vi "Set Drive Motors.vi"(5 "Disable":bool, 6 "Drive PID Slot":i32, 7 "Max Velocity(RPM)":dbl=200.0, 8 "Drive Control Mode":T11, 9 "Motor List":T1[](array[typedef])=[enum."Right-Front", enum."Left-Front", enum."Left-Back", enum."Right-Back"], 10 "Swerve Data":T2 {"Back Right"."Angle" scale format="%.3f"; "Back Right"."Velocity" scale=-1.0..1.0 scale format="%.1f"; "Back Left"."Angle" scale format="%.3f"; "Back Left"."Velocity" scale=-1.0..1.0 scale format="%.1f"; "Front Left"."Angle" scale format="%.3f"; "Front Left"."Velocity" scale=-1.0..1.0 scale format="%.1f"; "Front Right"."Angle" scale format="%.3f"; "Front Right"."Velocity" scale=-1.0..1.0 scale format="%.1f"}, 11 "Drive Refs":T6[](array[typedef])) -> (1 "Speeds":dbl[](array[numeric]), 3 "Array Out":T6[](array[typedef]))   [LabVIEW 2023, in "TShirtWork-SwerveDrive_ACT_ts.lvlib"]
uses:
  TShirtWork-SwerveDrive_ACT_ts.lvlib
  <vilib>/Rock Robotics/SystemInterfaces/DIO/FPGA_DIOPWMChannel.ctl
  <vilib>/Rock Robotics/WPI/PWM/WPI_PWMDeadband.ctl
  <vilib>/Rock Robotics/WPI/MotorControl/WPI_MotorControlType.ctl
  <vilib>/Rock Robotics/SystemInterfaces/DIO/FPGA_DIOChannel.ctl
  <vilib>/Rock Robotics/WPI/MotorControl/WPI_MotorControlDeviceRef.ctl
  <vilib>/Rock Robotics/WPI/ThirdParty/REV Robotics/REVLib/Typedef/Spark MAX Control Type.ctl
  Shared Code/TypeDefs/Level_Velocity plus-minus 1.ctl
  Shared Code/TypeDefs/Dial_Compase heading unit circle CCW positive.ctl
  Shared Code/TypeDefs/Cluster_Module Velocity-Direction-Rotations.ctl
  Shared Code/TypeDefs/Cluster_Swerve 4 Steer and Velocity.ctl
  Shared Code/TypeDefs/ENUM_Module Position.ctl
panel:
  # "\"Front\" of Robot"
  # "Right Hand Rule"
  # "X"
  # "+CCW"
  # "Y"
  # "(0,0)"
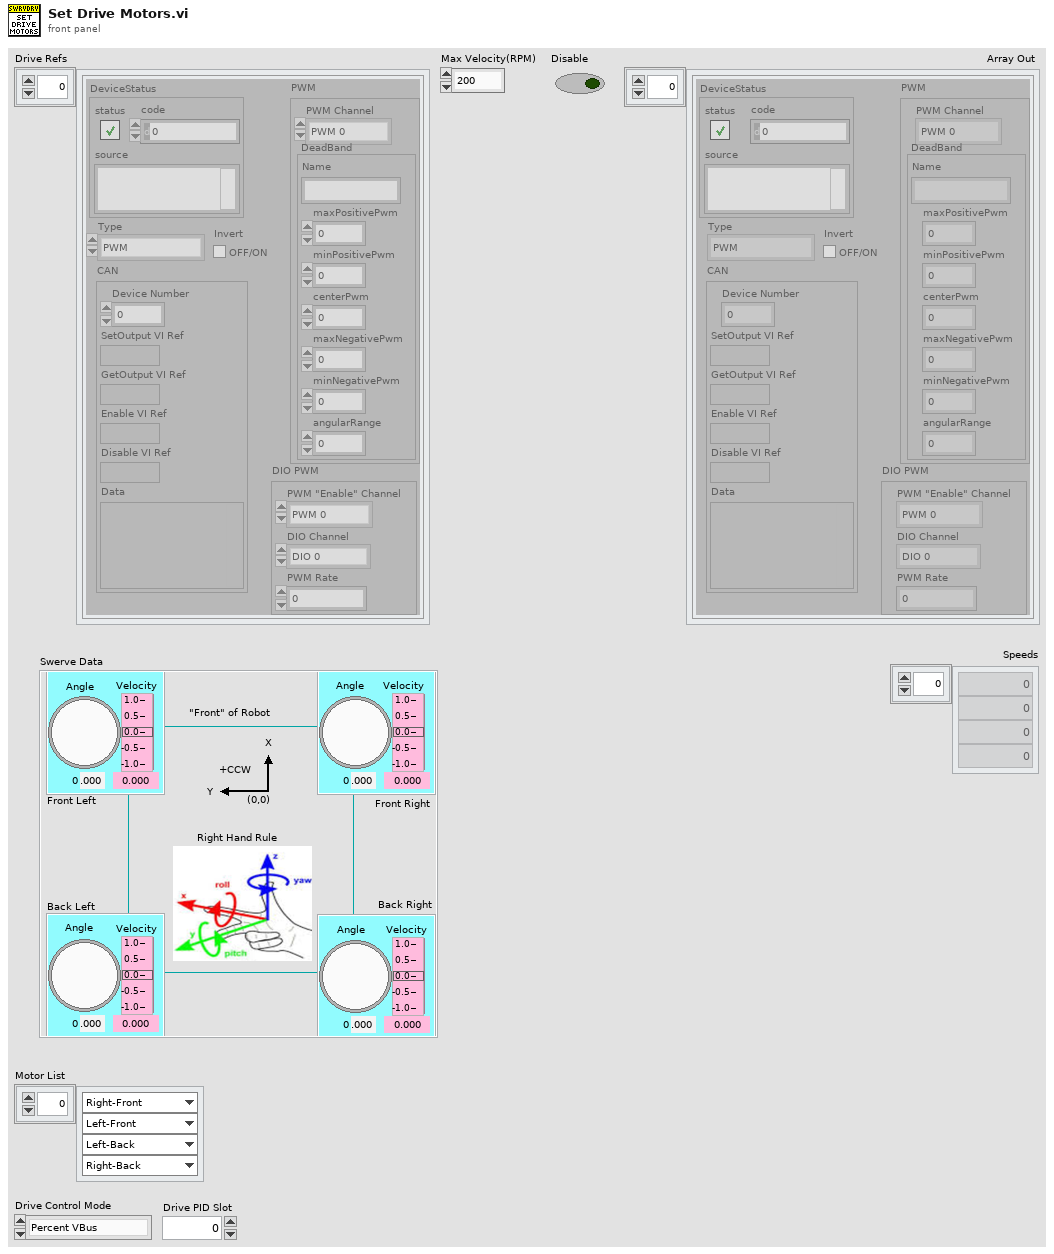
[diagram p1: front panel]
types:
  T1 = typedef "ENUM_Module Position.ctl" = enum16{"Left-Front", "Right-Front", "Left-Back", "Right-Back"}
  T2 = typedef "Cluster_Swerve 4 Steer and Velocity.ctl" = cluster{"Front Right":T3, "Front Left":T3, "Back Left":T3, "Back Right":T3}
  T3 = typedef "Cluster_Module Velocity-Direction-Rotations.ctl" = cluster{"Velocity":T4, "Angle":T5, "Rotations Count":dbl}
  T4 = typedef "Level_Velocity plus-minus 1.ctl" = dbl
  T5 = typedef "Dial_Compase heading unit circle CCW positive.ctl" = dbl
  T6 = typedef "WPI_MotorControlDeviceRef.ctl" = cluster{"DeviceStatus":errorcluster, "Type":T7, "PWM":cluster{"PWM Channel":T8, "DeadBand":T9}, "CAN":cluster{"Device Number":u8, "SetOutput VI Ref":variant, "GetOutput VI Ref":variant, "Enable VI Ref":variant, "Disable VI Ref":variant, "Data":variant}, "Invert":bool, "DIO PWM":cluster{"PWM \"Enable\" Channel":T8, "DIOChannel":T10, "PWM Rate":dbl}}
  T7 = typedef "WPI_MotorControlType.ctl" = enum16{"PWM", "CAN", "DIO PWM"}
  T8 = typedef "FPGA_DIOPWMChannel.ctl" = enum8{"PWM 0", "PWM 1", "PWM 2", "PWM 3", "PWM 4", "PWM 5", "PWM 6", "PWM 7", "PWM 8", "PWM 9", "PWM MXP 0", "PWM MXP 1", "PWM MXP 2", "PWM MXP 3", "PWM MXP 4", "PWM MXP 5", "PWM MXP 6", "PWM MXP 7", "PWM MXP 8", "PWM MXP 9", "Invalid"}
  T9 = typedef "WPI_PWMDeadband.ctl" = cluster{"Name":string, "maxPositivePwm":i32, "minPositivePwm":i32, "centerPwm":i32, "maxNegativePwm":i32, "minNegativePwm":i32, "angularRange":u16}
  T10 = typedef "FPGA_DIOChannel.ctl" = enum8{"DIO 0", "DIO 1", "DIO 2", "DIO 3", "DIO 4", "DIO 5", "DIO 6", "DIO 7", "DIO 8", "DIO 9", "DIO MXP 0", "DIO MXP 1", "DIO MXP 2", "DIO MXP 3", "DIO MXP 4", "DIO MXP 5", "DIO MXP 6", "DIO MXP 7", "DIO MXP 8", "DIO MXP 9", "DIO MXP 10", "DIO MXP 11", "DIO MXP 12", "DIO MXP 13", "DIO MXP 14", "DIO MXP 15", "SPI Port CS1", "SPI Port CS2", "SPI Port CS3", "SPI Port MISO", "SPI Port MOSI", "Invalid"}
  T11 = typedef "Spark MAX Control Type.ctl" = enum16{"Percent VBus", "Voltage", "Velocity", "Position", "Smart Motion", "Current", "Smart Velocity"}
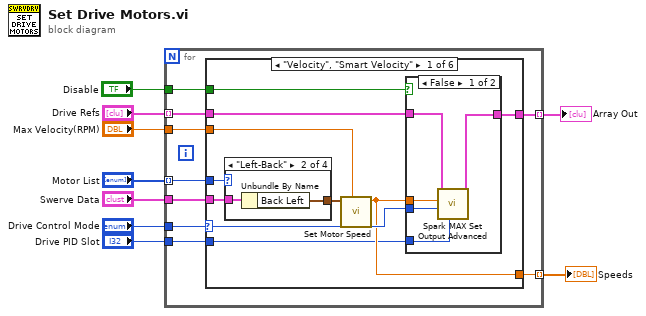
[diagram p0: block diagram]
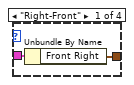
[diagram p3: hidden frame]
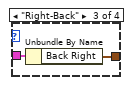
[diagram p4: hidden frame]
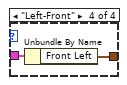
[diagram p5: hidden frame]
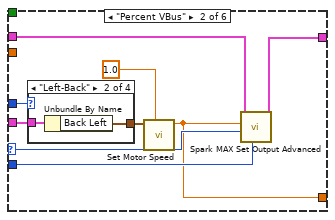
[diagram p6: hidden frame]
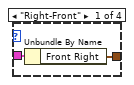
[diagram p7: hidden frame]
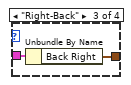
[diagram p8: hidden frame]
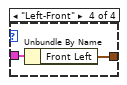
[diagram p9: hidden frame]
diagram:
  n1 = for {
    tunnel: "Drive Refs" -> [w18] mode=indexing
    tunnel: "Drive Control Mode" -> [w17]
    tunnel: "Drive PID Slot" -> [w16]
    tunnel: [w15] -> w9 mode=indexing
    tunnel: "Max Velocity(RPM)" -> [w12]
    tunnel: "Motor List" -> [w14] mode=indexing
    tunnel: "Swerve Data" -> [w13]
    tunnel: [w11] -> w2 mode=indexing
    tunnel: "Disable" -> [w10]
    n2 = case shown="\"Velocity\", \"Smart Velocity\"" w17 {
      selector: w17 -> [w27 w50 _ _ _ _]
      tunnel: w18 -> [w28 w51 w60 w61 w62 w63]
      tunnel: w16 -> [w20 w49 _ _ _ _]
      tunnel: [w26 w48 w60 w61 w62 w63] -> w15
      tunnel: w14 -> [w24 w46 _ _ _ _]
      tunnel: w13 -> [w25 w47 _ _ _ _]
      tunnel: w12 -> [w22 _ _ _ _ _]
      tunnel: [w21 w43 _ _ _ _] -> w11
      tunnel: w10 -> [w19 _ _ _ _ _]
      frame "Velocity", "Smart Velocity" {
        n3 = case shown="\"Left-Back\"" w24 {
          tunnel: w25 -> [w36 w38 w40 w42]
          tunnel: [w35 w37 w39 w41] -> w23
          frame "Right-Front" {
            n4 = Unbundle By Name(w36) -> ("Front Right"=w35:T3)
          }
          frame "Left-Back" {
            n5 = Unbundle By Name(w38) -> ("Back Left"=w37:T3)
          }
          frame "Right-Back" {
            n6 = Unbundle By Name(w40) -> ("Back Right"=w39:T3)
          }
          frame "Left-Front" {
            n7 = Unbundle By Name(w42) -> ("Front Left"=w41:T3)
          }
        }
        n8 = call "Set Motor Speed.vi"("Max Velocity"=w22, "Front Left"=w23) -> ("Velocity Value Set Out"=w21:dbl)  [unwired: 9 in]
        n9 = case shown="False" w19 {
          tunnel: w28 -> [w33 w34]
          tunnel: w27 -> [w32 _]
          tunnel: [w31 w34] -> w26
          tunnel: w21 -> [w30 _]
          tunnel: w20 -> [w29 _]
          frame False {
            n10 = call <vilib>:"Spark MAX Set Output Advanced.vi"("PIDF Slot (0)"=w29, "Control Mode"=w32, "Setpoint"=w30, "MotorControlDevRef"=w33) -> ("MotorControlDevRef"=w31:T6)  [unwired: 6 in, 1 out]
          }
          frame True {
          }
        }
      }
      frame "Percent VBus" {
        n11 = case shown="\"Left-Back\"" w46 {
          tunnel: w47 -> [w53 w55 w57 w59]
          tunnel: [w52 w54 w56 w58] -> w45
          frame "Right-Front" {
            n12 = Unbundle By Name(w53) -> ("Front Right"=w52:T3)
          }
          frame "Left-Back" {
            n13 = Unbundle By Name(w55) -> ("Back Left"=w54:T3)
          }
          frame "Right-Back" {
            n14 = Unbundle By Name(w57) -> ("Back Right"=w56:T3)
          }
          frame "Left-Front" {
            n15 = Unbundle By Name(w59) -> ("Front Left"=w58:T3)
          }
        }
        n16 = call "Set Motor Speed.vi"("Max Velocity"=1.0, "Front Left"=w45) -> ("Velocity Value Set Out"=w43:dbl)  [unwired: 9 in]
        n17 = call <vilib>:"Spark MAX Set Output Advanced.vi"("PIDF Slot (0)"=w49, "Control Mode"=w50, "Setpoint"=w43, "MotorControlDevRef"=w51) -> ("MotorControlDevRef"=w48:T6)  [unwired: 6 in, 1 out]
      }
      frame "Current" {
      }
      frame "Voltage" {
      }
      frame "Position" {
      }
      frame "Smart Motion" {
      }
    }
  }
  "Array Out" <- w9
  "Speeds" <- w2
